vi "Get All Messages.vi"(5 "delete from server (Y)?":bool=TRUE, 7 "error in":errorcluster, 8 "POP server name/IP":string, 9 "password":string, 10 "username":string) -> (0 "error out":errorcluster, 2 "Message Summary":string="\r\n", 3 "message array":string[](array[string]))   [LabVIEW 2012]
doc: "This high-level VI queries a POP mail server to see if there are any new messages waiting to be read, then retrieves each message that it finds.\n\nBy default, mails are deleted from the server after they are retrieved, but you can specify not to delete the messages, leaving them on the server for future use.\n\nUsername, password, and POP server name must be valid identifiers associated with an ISP account or other POP mail service."
panel:
  out "Downloading Message#:":i32
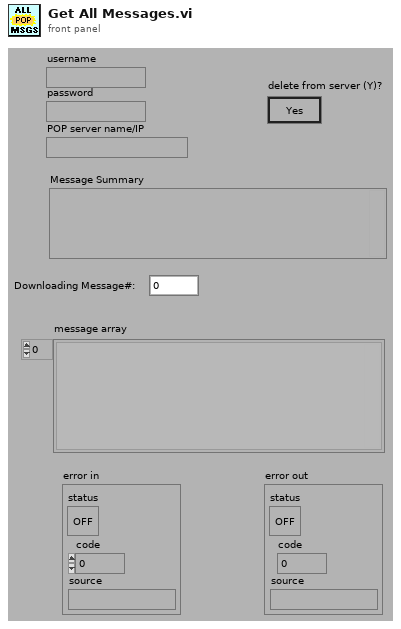
[diagram p1: front panel]
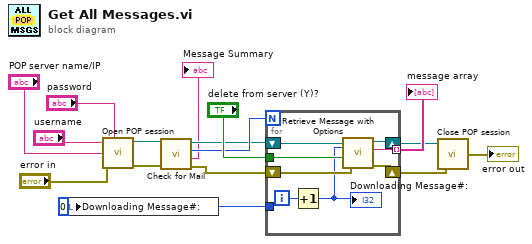
[diagram p0: block diagram]
diagram:
  w2 = 0 ("Downloading Message#:")
  n1 = local write "Downloading Message#:"(w2) -> ()
  n2 = call "Open POP session.vi"("username"="username", "password"="password", "POP server name/IP"="POP server name/IP", "error in"="error in") -> ("connection ID out"=w12:refnum<k5>, "error out"=w11:errorcluster)  [unwired: 2 in, 1 out]
  n3 = call "Check for Mail.vi"("error in"=w11, "connection ID in"=w12) -> ("error out"=w9:errorcluster, "LIST response"=→"Message Summary":string, "# messages"=w10:i32, "connection ID out"=w7:refnum<k5>)  [unwired: 2 in]
  n4 = for {
    N: w10 -> [_]
    shift-right: [w20] -> w5
    shift-left: w9 -> [w23]
    tunnel: "delete from server (Y)?" -> [w24]
    tunnel: [w19] -> w8 mode=indexing
    shift-right: [w17] -> w6
    shift-left: w7 -> [w18]
    tunnel: w2 -> [_]
    i -> [w22]
    n5 = Increment(x=w22) -> (x+1=w21:i32)
    "Downloading Message#:" <- w21
    n6 = call "Retrieve Message with Options.vi"("error in"=w23, "delete from server (Y)?"=w24, "message #"=w21, "connection ID in"=w18) -> ("error out"=w20:errorcluster, "Message"=w19:string, "connection ID out"=w17:refnum<k5>)  [unwired: 1 in]
  }
  "message array" <- w8
  n7 = call "Close POP session.vi"("error in (no error)"=w5, "connection ID"=w6) -> ("error out"=→"error out":errorcluster)
